vi "Read pitches.vi"(8 "error in (no error)":errorcluster, 11 "OWIS_TANGO in":refnum<class "OWIS_TANGO.lvclass">) -> (0 "error out":errorcluster, 2 "pitches":dbl[](array[numeric]), 3 "OWIS_TANGO out":refnum<class "OWIS_TANGO.lvclass">)   [LabVIEW 2020, in "OWIS_TANGO.lvclass"]
uses:
  OWIS_TANGO.lvclass
  DelayLine.lvclass
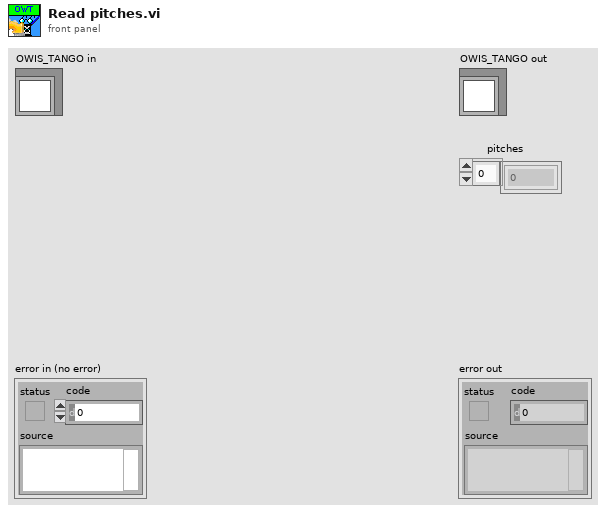
[diagram p1: front panel]
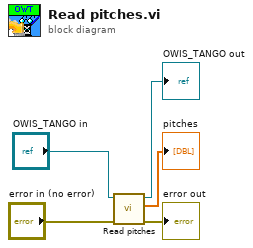
[diagram p0: block diagram]
diagram:
  n1 = call-parent "Read pitches.vi"("error in (no error)"="error in (no error)", "DelayLine in"="OWIS_TANGO in") -> ("error out"=→"error out":errorcluster, "pitches"=→"pitches":dbl[], "DelayLine out"=→"OWIS_TANGO out":refnum<class "OWIS_TANGO.lvclass">)  [unwired: 7 in]
